vi "Add Rx Label.vi"(6 "create channels":T1, 8 "error in":errorcluster, 9 "SDI value":T3=-1 items=["All"=-1, "0 (b00)"=0, "1 (b01)"=1, "2 (b10)"=2, "3 (b11)"=3], 10 "label value":u32, 11 "port in":T2 format="%.0x") -> (0 "error out":errorcluster, 2 "label":T2 format="%.0x", 3 "port out":T2 format="%.0x")   [LabVIEW 2020, in "AIM ARINC 429 Scripting.lvlib"]
doc: "Adds an Rx label to the specified incoming (Rx) port. Returns the newly added <b>label</b> reference."
uses:
  AIM ARINC 429 Scripting.lvlib
  Shared/SDI.ctl
  <vilib>/NI VeriStand/Custom Device API/Custom Device Item Ref.ctl
  Shared/Label Properties.ctl
  Shared/Label.ctl
  <vilib>/NI VeriStand/Custom Device API/Custom Device Channel.ctl
  <vilib>/NI VeriStand/Custom Device API/Custom Device Channel Type.ctl
  Constants.vi
  ARINC 429/Constants.vi
  <vilib>/NI VeriStand/Custom Device API/Custom Device API.lvlib
  ARINC 429/ARINC 429 Scripting.lvlib
  Import/ARINC 429 Import.lvlib
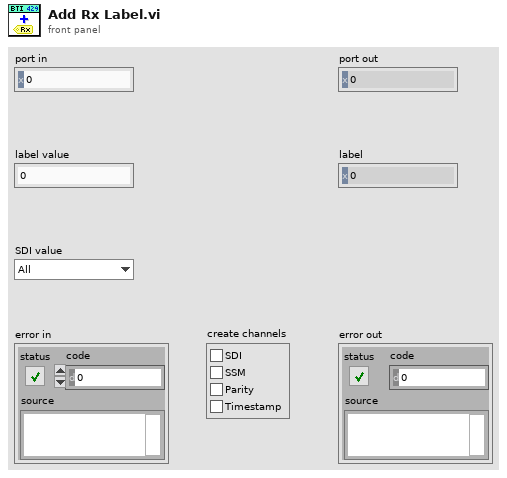
[diagram p1: front panel]
types:
  T1 = cluster{"SDI":bool, "SSM":bool, "Parity":bool, "Timestamp":bool}
  T2 = typedef "Custom Device API.lvlib/Custom Device Item Ref.ctl" = u64
  T3 = typedef "SDI.ctl" = i32
  T4 = typedef "Direction.ctl" = enum16{"Rx", "Tx"}
  T5 = typedef "Custom Device API.lvlib/Custom Device Channel.ctl" = cluster{"Type":T6, "Units":string, "Default Value":dbl, "Faultable":bool, "Scalable":bool}
  T6 = typedef "Custom Device API.lvlib/Custom Device Channel Type.ctl" = enum16{"Input", "Output"}
  T7 = typedef "Label Properties.ctl" = cluster{"label (Dec)":T8, "SDI value":u8, "SDI enabled":bool}
  T8 = typedef "Label.ctl" = u8
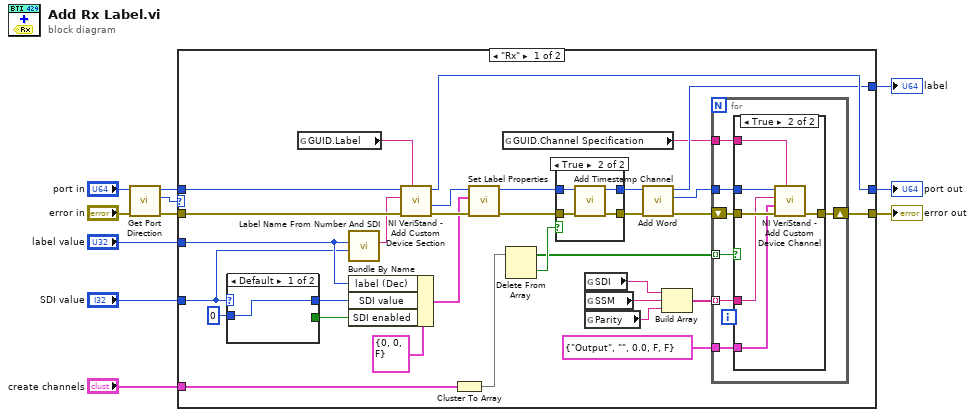
[diagram p0: block diagram]
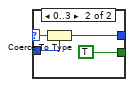
[diagram p4: hidden frame]
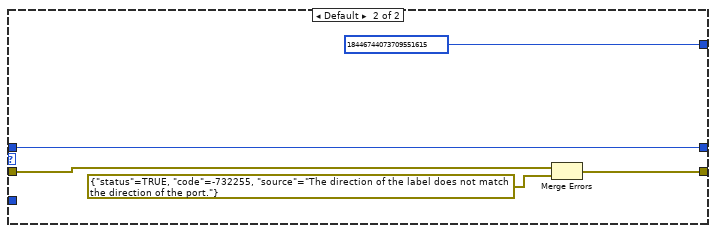
[diagram p5: hidden frame]
diagram:
  n1 = call "Get Port Direction.vi"("error in"="error in", "port ref in"="port in") -> ("error out"=w8:errorcluster, "direction"=w1:T4, "port ref out"=w9:T2)  [unwired: 7 in]
  n2 = case shown="\"Rx\"" w1 {
    tunnel: w9 -> [w35 w73]
    tunnel: w8 -> [w34 w71]
    tunnel: [w31 w73] -> w7
    tunnel: "label value" -> [w28 _]
    tunnel: "SDI value" -> [w26 _]
    tunnel: "create channels" -> [w25 _]
    tunnel: [w22 T2 18446744073709551615 ("label ref out")] -> w3
    tunnel: [w20 w70] -> w2
    frame "Rx" {
      n3 = case shown="Default" w26 {
        selector: w26 -> [_ w68]
        tunnel: [w64 w65] -> w27
        tunnel: u8 0 ("SDI value") -> [w64 w67]
        tunnel: [_ TRUE] -> w32
        frame Default {
        }
        frame 0..3 {
          n4 = Coerce To Type(0:w68, 1:w67) -> (2:w65:u8)
        }
      }
      n5 = global read "Constants.vi" "GUID.Label"() -> (w38:string)
      n6 = call "Label Name From Number And SDI.vi"("SDI value"=w26, "label (Dec)"=w28) -> ("label name"=w29:string)  [unwired: 9 in]
      n7 = Bundle By Name(cluster=T7 {"label (Dec)"=0, "SDI value"=0, "SDI enabled"=FALSE} ("label properties"), "label (Dec)"=w28, "SDI value"=w27, "SDI enabled"=w32) -> (w36:T7)
      n8 = call <vilib>:"NI VeriStand - Add Custom Device Section.vi"("GUID (Default Section)"=w38, "error in (no error)"=w34, "Section Name"=w29, "Parent Ref in"=w35) -> ("error out"=w40:errorcluster, "Section Ptr"=w39:T2, "Parent Ref out"=w31:T2)  [unwired: 4 in, 1 out]
      n9 = Cluster To Array(cluster=w25) -> (array=w24:bool[])
      n10 = call "Set Label Properties.vi"("error in"=w40, "label properties"=w36, "label ref"=w39) -> ("error out"=w41:errorcluster, "label ref out"=w30:T2)  [unwired: 7 in]
      n11 = global read "Constants.vi" "GUID.Channel Specification"() -> (w17:string)
      n12 = Delete From Array(array=w24) -> (deleted portion=w23:bool, array with subset deleted=w19:bool[])  [unwired: 2 in]
      n13 = case shown="True" w23 {
        tunnel: [w59 w63] -> w43
        tunnel: [w58 w62] -> w42
        tunnel: w41 -> [w58 w61]
        tunnel: w30 -> [w59 w60]
        frame False {
        }
        frame True {
          n14 = call "Add Timestamp Channel.vi"("error in"=w61, "label ref"=w60) -> ("error out"=w62:errorcluster, "label ref out"=w63:T2)  [unwired: 8 in]
        }
      }
      n15 = global read "Constants.vi" "SDI"() -> (w14:string)
      n16 = global read "Constants.vi" "SSM"() -> (w15:string)
      n17 = global read "Constants.vi" "Parity"() -> (w13:string)
      n18 = call "Add Word.vi"("error in"=w42, "label ref"=w43) -> ("error out"=w21:errorcluster, "word ref"=w18:T2, "label ref out"=w22:T2)  [unwired: 6 in, 1 out]
      n19 = Build Array(w14, w15, w13) -> (w12:string[])
      n20 = for {
        shift-right: [w49] -> w20
        shift-left: w21 -> [w48]
        tunnel: w19 -> [w50] mode=indexing
        tunnel: w18 -> [w47]
        tunnel: w17 -> [w46]
        tunnel: T5 {"Type"=enum."Output", "Units"="", "Default Value"=0.0, "Faultable"=FALSE, "Scalable"=FALSE} ("Channel") -> [w45]
        tunnel: w12 -> [w44] mode=indexing
        n21 = case shown="True" w50 {
          tunnel: [w51 w57] -> w49
          tunnel: w48 -> [w51 w56]
          tunnel: w47 -> [_ w53]
          tunnel: w46 -> [_ w55]
          tunnel: w45 -> [_ w54]
          tunnel: w44 -> [_ w52]
          frame False {
          }
          frame True {
            n22 = call <vilib>:"NI VeriStand - Add Custom Device Channel.vi"("GUID (Default Channel)"=w55, "error in (no error)"=w56, "Channel"=w54, "Channel Name"=w52, "Parent Ref in"=w53) -> ("error out"=w57:errorcluster)  [unwired: 3 in, 3 out]
          }
        }
      }
    }
    frame Default {
      n23 = Merge Errors(w71, errorcluster {"status"=TRUE, "code"=-732255, "source"="The direction of the label does not match the direction of the port."} ("error in")) -> (w70:errorcluster)
    }
  }
  "label" <- w3
  "error out" <- w2
  "port out" <- w7
